vi "Validate Path Length.vi"(8 "error in (no error)":errorcluster, 11 "Path in":path) -> (0 "error out":errorcluster, 3 "Path out":path)   [LabVIEW 2019, in "gRPC Scripting Tools.lvlib"]
doc: "Check if the path given exceeds platform-specific maximum lengths for either path length or filename length."
uses:
  gRPC Scripting Tools.lvlib
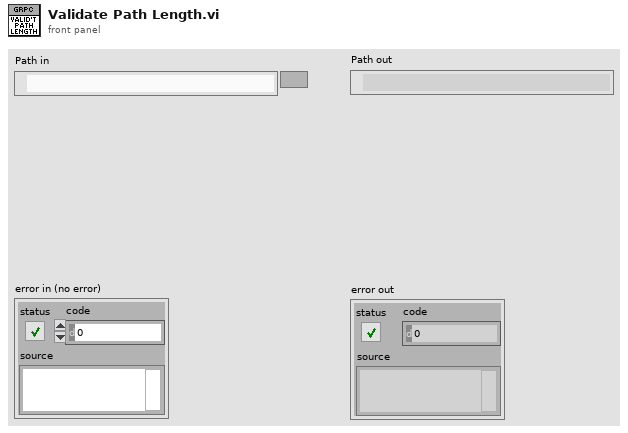
[diagram p1: front panel]
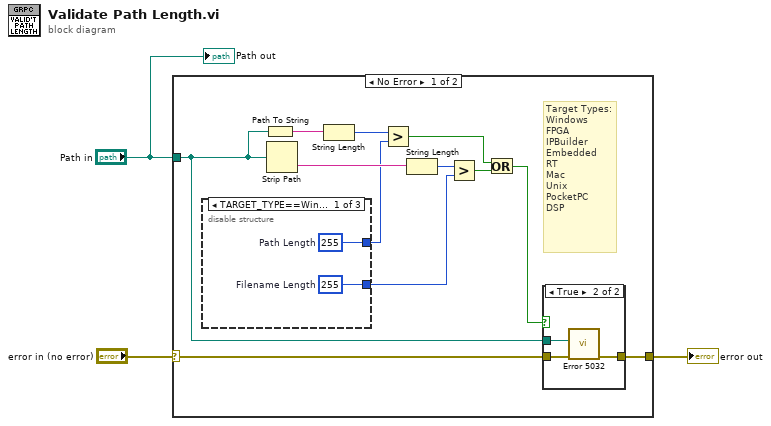
[diagram p0: block diagram]
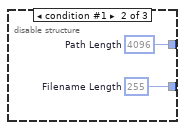
[diagram p2: hidden frame]
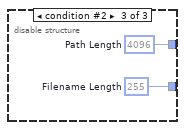
[diagram p3: hidden frame]
diagram:
  n1 = case shown="No Error" "error in (no error)" {
    selector: "error in (no error)" -> [w6 w26]
    tunnel: "Path in" -> [w4 _]
    tunnel: [w5 w26] -> w1
    frame No Error {
      # "Target Types:\nWindows\nFPGA\nIPBuilder\nEmbedded\nRT\nMac\nUnix\nPocketPC\nDSP"
      n2 = disable-structure shown="TARGET_TYPE==Windows" {
        disable-tunnel: [w17 w19 w21] -> w10
        disable-tunnel: [w16 w18 w20] -> w13
        frame condition #0 (active) {
          w16 = 255  # Filename Length
          w17 = 255  # Path Length
        }
        frame condition #1 {
          w18 = 255  # Filename Length
          w19 = 4096  # Path Length
        }
        frame condition #2 {
          w20 = 255  # Filename Length
          w21 = 4096  # Path Length
        }
      }
      n3 = Path To String(path=w4) -> (string=w12:string)
      n4 = Strip Path(path=w4) -> (name=w15:string)  [unwired: 1 out]
      n5 = String Length(string=w12) -> (length=w11:i32)
      n6 = Greater?(x=w11, y=w10) -> (0:w9:bool)
      n7 = String Length(string=w15) -> (length=w14:i32)
      n8 = Greater?(x=w14, y=w13) -> (0:w8:bool)
      n9 = Or(x=w9, y=w8) -> (x .or. y?=w7:bool)
      n10 = case shown="True" w7 {
        tunnel: w6 -> [w22 w25]
        tunnel: [w22 w24] -> w5
        tunnel: w4 -> [_ w23]
        frame False {
        }
        frame True {
          n11 = call "Error 5032.vi"("error in (no error)"=w25, "Path"=w23) -> ("error out"=w24:errorcluster)  [unwired: 9 in]
        }
      }
    }
    frame Error {
    }
  }
  "error out" <- w1
  "Path out" <- "Path in"
